vi "Double move fwd PID with average.vi"(0 "Distance":dbl, 1 "Gains":T1={"proportional gain (Kc)"=1.0, "integral time (Ti, min)"=0.01, "derivative time (Td, min)"=0.0} {"derivative time (Td, min)" format="%.3f"; "integral time (Ti, min)" format="%.3f"; "proportional gain (Kc)" format="%.3f"}, 3 "Range":cluster{"output high":dbl, "output low":dbl}={"output high"=1.0, "output low"=0.0} {"output low" format="%.2f"; "output high" format="%.2f"}, 5 "Encoder Left":dbl, 9 "Encoder Right":dbl, 11 "Precision":dbl=0.5 format="%#_13g", 12 "Loop Timer":i32=20, 13 "Soft start":dbl=1.0, 14 "Time to stop":i32=300) -> (4 "PWM out":dbl=0.5 format="%#_13g", 15 "finished?":bool)   [LabVIEW 2017]
panel:
  # "Time to stop - Tempo que o encoder deve retornar um valor dentro do range da precision para a função considerar que o sistema está parado.\n\nDistance - Setpoint em unidades do encoder.\n\nLoop Timer - Tempo de iteração do loop em que a função está.\n\nPrecision - Range que a função considera \"close enough\" ao setpoint.\n\nEncoder Right - Valor atual do encoder da direita.\n\nEncoder Left - Valor atual do encoder da esquerda\n\nGains - Ganhos do PID.\n\nRange - limite superior e inferior do PID.\n\nSoft Start - constante que aumenta ou diminui o tempo de aceleração no início do movimento"
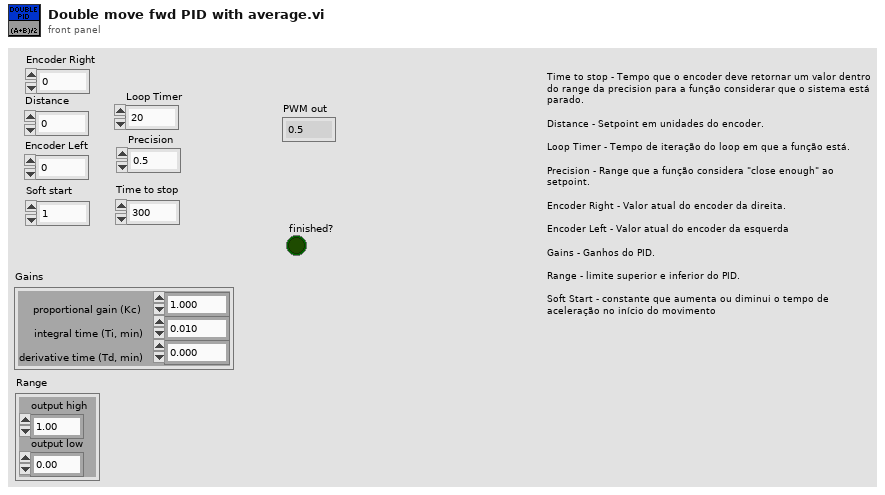
[diagram p1: front panel]
types:
  T1 = cluster{"proportional gain (Kc)":dbl, "integral time (Ti, min)":dbl, "derivative time (Td, min)":dbl}
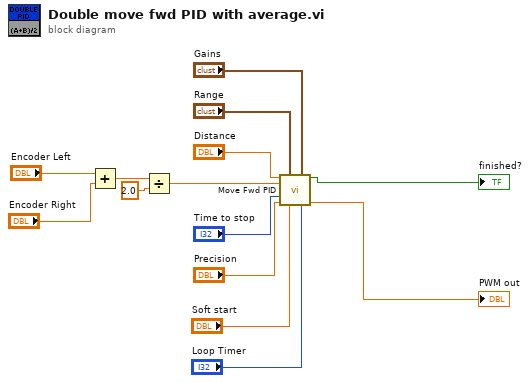
[diagram p0: block diagram]
diagram:
  n1 = Add(x="Encoder Left", y="Encoder Right") -> (x+y=w4:dbl)
  n2 = Divide(x=w4, y=2.0) -> (x/y=w2:dbl)
  n3 = call "Move Fwd PID.vi"("Distance"="Distance", "Range"="Range", "Gains"="Gains", "Encoder Count"=w2, "Time to stop"="Time to stop", "Precision"="Precision", "Soft start"="Soft start", "Loop Timer"="Loop Timer") -> ("Finished?"=→"finished?":bool, "Output"=→"PWM out":dbl)  [unwired: 6 in]
